vi "Waveform to XY (single).vi"(8 "error in (no error)":errorcluster, 11 "Waveform in":waveform(dbl)) -> (0 "error out":errorcluster, 3 "XY-data out":cluster{"X-array":dbl[], "Y-array":dbl[]} {"Y-array" format="%.2p"; "X-array" format="%.2p"})   [LabVIEW 2019, in "xy_utilities.lvlib"]
doc: "Convert <b>Waveform</b> to <b>XY-data</b>"
uses:
  xy_utilities.lvlib
  <vilib>/Waveform/WDTOps.llb/WDT Waveform to XY Pairs DBL.vi
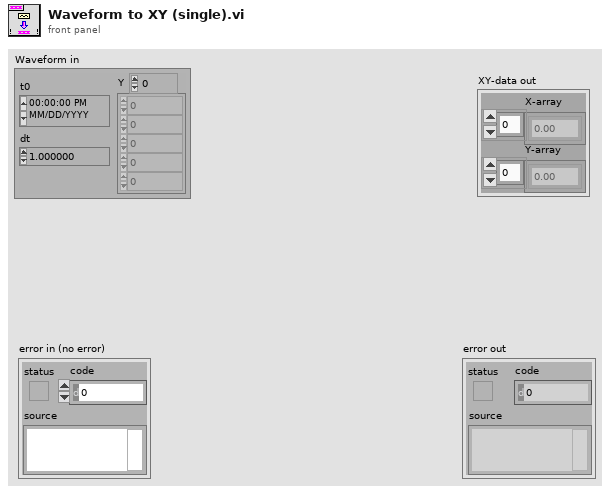
[diagram p1: front panel]
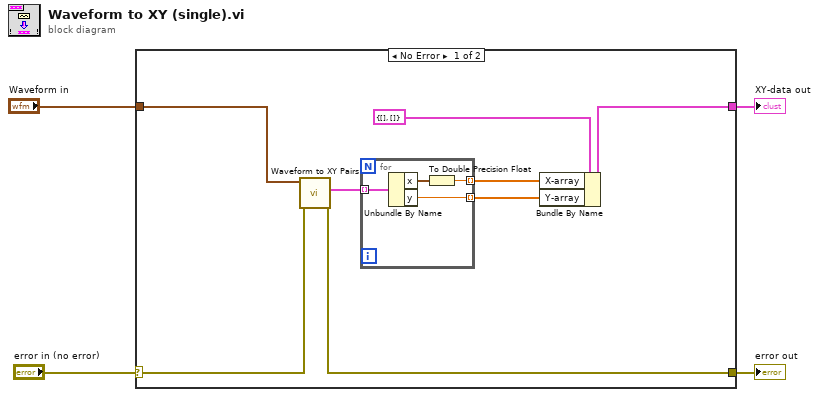
[diagram p0: block diagram]
diagram:
  n1 = case shown="No Error" "error in (no error)" {
    selector: "error in (no error)" -> [w8 w17]
    tunnel: [w7 w17] -> w3
    tunnel: "Waveform in" -> [w9 _]
    tunnel: [w12 _] -> w1
    frame No Error {
      n2 = call-poly <vilib>:"Waveform to XY Pairs.vi"("error in (no error)"=w8, "waveform in"=w9) -> ("error out"=w7:errorcluster, "XY pairs"=w11:cluster{"x":timestamp, "y":dbl}[])  [unwired: 7 in, 1 out]
      n3 = for {
        tunnel: w11 -> [w16] mode=indexing
        tunnel: [w13] -> w6 mode=indexing
        tunnel: [w14] -> w5 mode=indexing
        n4 = Unbundle By Name(w16) -> ("x"=w15:timestamp, "y"=w14:dbl)
        n5 = To Double Precision Float(number=w15) -> (double precision float=w13:dbl)
      }
      n6 = Bundle By Name(cluster=cluster{"X-array":dbl[], "Y-array":dbl[]} {"X-array"=[], "Y-array"=[]} ("XY-data out"), "X-array"=w6, "Y-array"=w5) -> (w12:cluster{"X-array":dbl[], "Y-array":dbl[]})
    }
    frame Error {
    }
  }
  "error out" <- w3
  "XY-data out" <- w1
